vi "RTFIFO test.vi"() -> ()   [LabVIEW 2014]
uses:
  <vilib>/Platform/TimedLoop/XDataNode/timing_clust.ctl
  <vilib>/Platform/TimedLoop/XDataNode/nitl_modes.ctl
  <vilib>/Platform/TimedLoop/XDataNode/wakeup.ctl
  <vilib>/Platform/TimedLoop/XDataNode/XDataNode.xnode
  <vilib>/Platform/TimedLoop/XDataNode/XDNodeRunTimeDep.lvlib
panel:
  out "Numeric 1":i32
  out "Numeric 2":i32
  out "Update 3":u32
  out "Update 2":u32
  out "Update1":u32
  out "stop":bool
  in  "Array":i32[](array[numeric])
  out "element in":i32
  out "element out 2":i32
  out "element out":i32
  # "@1Hz"
  # "@5 Hz"
  # "@1Hz"
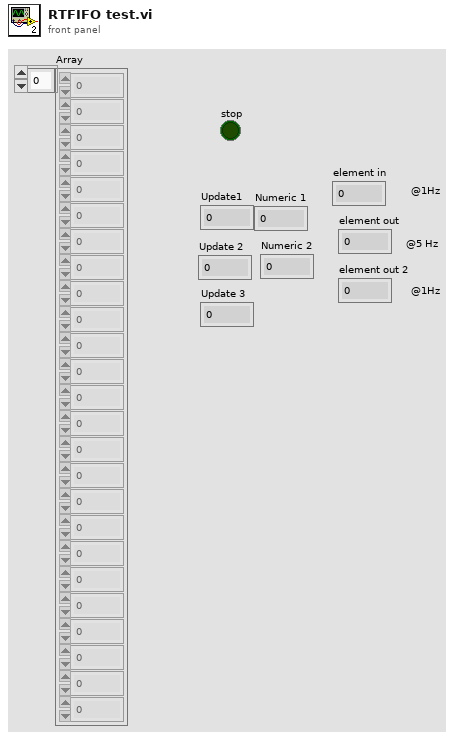
[diagram p1: front panel]
types:
  T1 = typedef "XDNodeRunTimeDep.lvlib/timing_clust.ctl" = cluster{"Expected End [f-1]":u64, "Actual End [f-1]":u64, "Finished Late? [f-1]":bool, "Expected End [i-1]":u64, "Actual End [i-1]":u64, "Finished Late? [i-1]":bool, "Expected Start [i]":u64, "Actual Start [i]":u64, "Expected Start [f]":u64, "Actual Start [f]":u64, "Source Name":string, "Structure Name":string, "Period":i64, "Deadline":i64, "Offset":i64, "Start":i64, "Priority":i32, "Timeout":i32, "Mode":T2, "Wakeup Reason":T3, "Error":errorcluster, "Source Type":string, "Secondary Source Type":string, "Global End Time":u64, "Global Start Time":u64, "Frame Duration":u64, "Iteration Duration":u64, "Assigned CPU":i32, "I/O Scan Engine Mode":u32}
  T2 = typedef "XDNodeRunTimeDep.lvlib/nitl_modes.ctl" = enum32{"No Change", "Process missed periods, maintain original phase", "Discard missed periods, maintain original phase", "Process missed periods, ignore original phase", "Discard missed periods, ignore original phase"}
  T3 = typedef "XDNodeRunTimeDep.lvlib/wakeup.ctl" = enum32{"Normal", "Aborted", "Asynchronous wakeup", "Timing source error", "Timed loop error", "Timeout"}
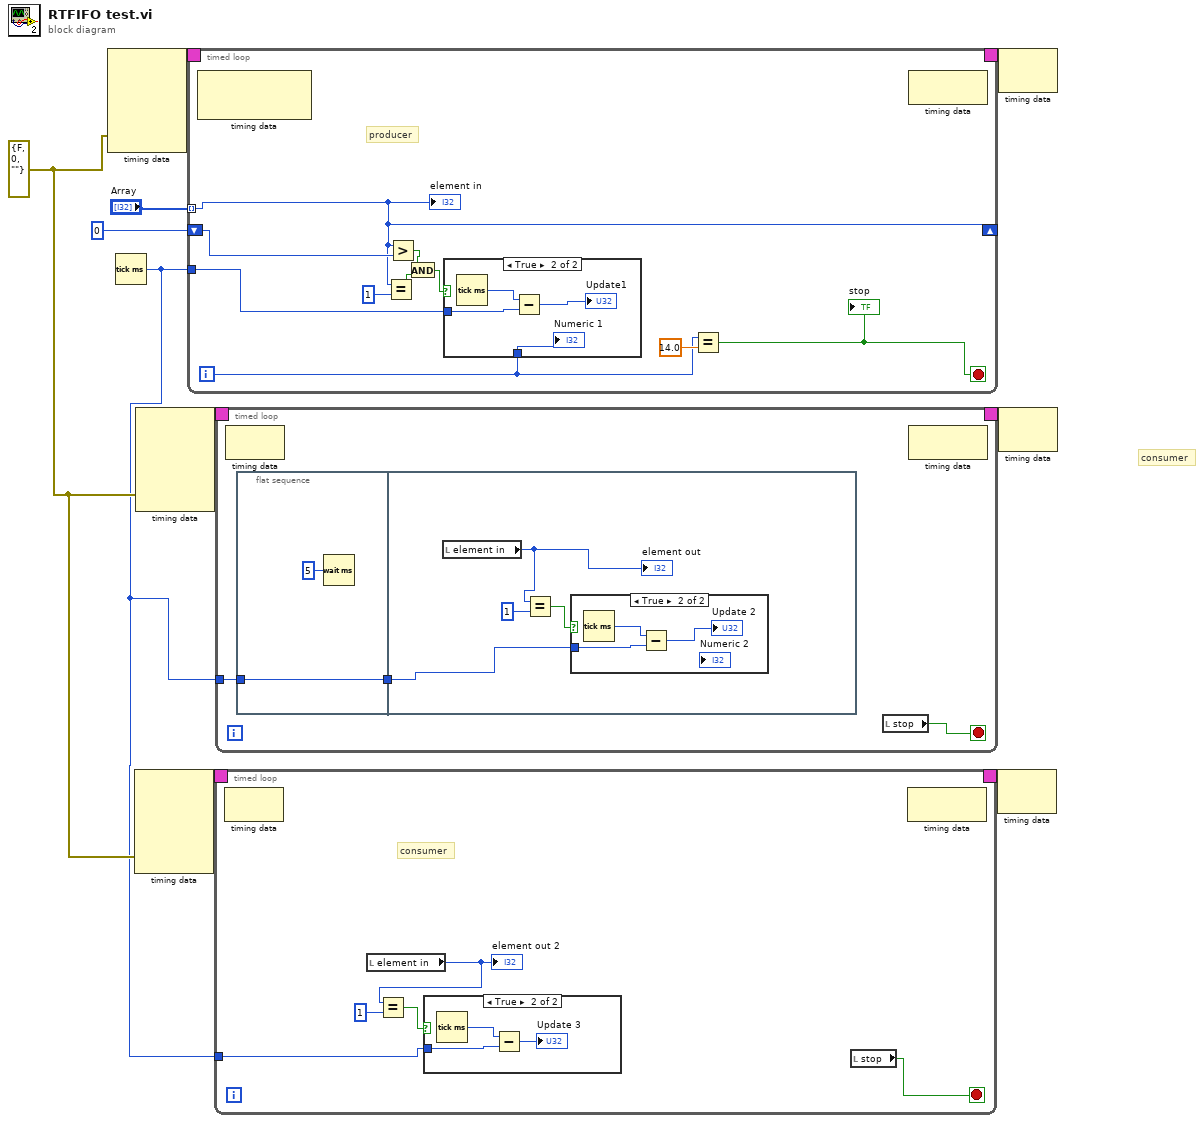
[diagram p0: block diagram]
diagram:
  w4 = errorcluster {"status"=FALSE, "code"=0, "source"=""} ("Error")
  # "consumer"
  n1 = node-c288(w4) -> (w10:T1)  [unwired: 4 in]
  n2 = Tick Count (ms)() -> (millisecond timer value=w2:u32)
  n3 = node-c288(w4) -> (w6:T1)  [unwired: 4 in]
  n4 = node-c288(w4) -> (w8:T1)  [unwired: 4 in]
  n5 = timed-loop {
    timing: w10 -> [_]
    timing-out: [_] -> w9
    tunnel: "Array" -> [w15] mode=indexing
    tunnel: w2 -> [w18]
    shift-right: [w15] -> _
    shift-left: 0 -> [w16]
    i -> [w17]
    stop <- w19 stop-if-true
    # "producer"
    n6 = node-c288() -> ()  [unwired: 1 in, 2 out]
    n7 = Equal?(x=w15, y=1) -> (x = y?=w13:bool)
    n8 = Greater?(x=w15, y=w16) -> (0:w12:bool)
    n9 = And(x=w12, y=w13) -> (x .and. y?=w11:bool)
    n10 = case shown="True" w11 {
      tunnel: w18 -> [_ w23]
      tunnel: w17 -> [_ w21]
      frame False {
      }
      frame True {
        n11 = Tick Count (ms)() -> (millisecond timer value=w24:u32)
        n12 = Subtract(x=w24, y=w23) -> (x-y=→"Update1":u32)
        "Numeric 1" <- w21
      }
    }
    n13 = Equal?(x=w17, y=14.0) -> (x = y?=w19:bool)
    "stop" <- w19
    n14 = node-c288() -> ()  [unwired: 1 in, 1 out]
    "element in" <- w15
  }
  n15 = timed-loop {
    timing: w6 -> [_]
    timing-out: [_] -> w5
    tunnel: w2 -> [w27]
    stop <- w31 stop-if-true
    # "consumer"
    n16 = node-c288() -> ()  [unwired: 1 in, 1 out]
    n17 = local read "element in"() -> (w28:i32)
    "element out 2" <- w28
    n18 = Equal?(x=w28, y=1) -> (x = y?=w30:bool)
    n19 = case shown="True" w30 {
      tunnel: w27 -> [_ w33]
      frame False {
      }
      frame True {
        n20 = Tick Count (ms)() -> (millisecond timer value=w34:u32)
        n21 = Subtract(x=w34, y=w33) -> (x-y=→"Update 3":u32)
      }
    }
    n22 = local read "stop"() -> (w31:bool)
    n23 = node-c288() -> ()  [unwired: 1 in, 1 out]
  }
  n24 = timed-loop {
    timing: w8 -> [_]
    timing-out: [_] -> w7
    tunnel: w2 -> [w37]
    stop <- w39 stop-if-true
    n25 = node-c288() -> ()  [unwired: 1 in, 1 out]
    n26 = flat-sequence {
      tunnel: [w40] -> w38
      tunnel: w37 -> [w40]
      tunnel: w38 -> [w42]
      frame #0 {
        n27 = Wait (ms)(milliseconds to wait=u32 5) -> ()  [unwired: 1 out]
      }
      frame #1 {
        n28 = local read "element in"() -> (w44:i32)
        "element out" <- w44
        n29 = Equal?(x=w44, y=1) -> (x = y?=w43:bool)
        n30 = case shown="True" w43 {
          tunnel: w42 -> [_ w47]
          frame False {
          }
          frame True {
            n31 = Tick Count (ms)() -> (millisecond timer value=w48:u32)
            n32 = Subtract(x=w48, y=w47) -> (x-y=→"Update 2":u32)
          }
        }
      }
    }
    n33 = local read "stop"() -> (w39:bool)
    n34 = node-c288() -> ()  [unwired: 1 in, 1 out]
  }
  n35 = node-c288(w5) -> ()  [unwired: 1 out]
  n36 = node-c288(w9) -> ()  [unwired: 1 out]
  n37 = node-c288(w7) -> ()  [unwired: 1 out]
